vi "PH_O2_Watch.publish State.vi"(0 "i ref in":refnum<vi>, 5 "error in (no error)":errorcluster) -> (14 "i ref out":refnum<vi>, 19 "error out":errorcluster)   [LabVIEW 2014, in "PH_O2_Watch.lvlib"]
doc: "By this VI the device state is published via DIM service\n\nno info (0): no failure, prealert or alert, but at least one tag without info\non (2): no failure, prealert or alert, no limit set (\"99%\")\nfailure (3): failure\nalam (4): no failure, but alert\nStatus 1 (5): no alert or failure, but prealert\nStatus 2 (6): no failure, prealert or alert, and concentration smaller or equal than limit\nStatus 3 (7): no failure, prealert or alert, and concentration grater than limit"
uses:
  PH_O2_Watch.lvlib
  PH_Basics/PH_StatusHandler/PH_StatusHandler.Status.ctl
  PH_Basics/PH_StatusHandler/PH_StatusHandler.lvlib
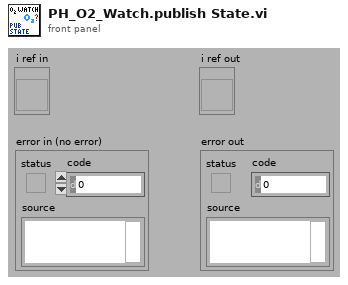
[diagram p1: front panel]
types:
  T1 = typedef "PH_StatusHandler.lvlib/PH_StatusHandler.Status.ctl" = i16
  T2 = typedef "PH_O2_Watch.lvlib/PH_O2_Watch.i attribute.ctl" = cluster{"GUI Refs":cluster{"PreAlert":refnum<vi>, "Alert":refnum<vi>, "Failure":refnum<vi>, "Concentration":refnum<vi>, "Delete":refnum<vi>, "Limit":refnum<vi>}, "State PreAlert":T1, "State Alert":T1, "State Failure":T1, "Concentration":dbl, "Limit":dbl}
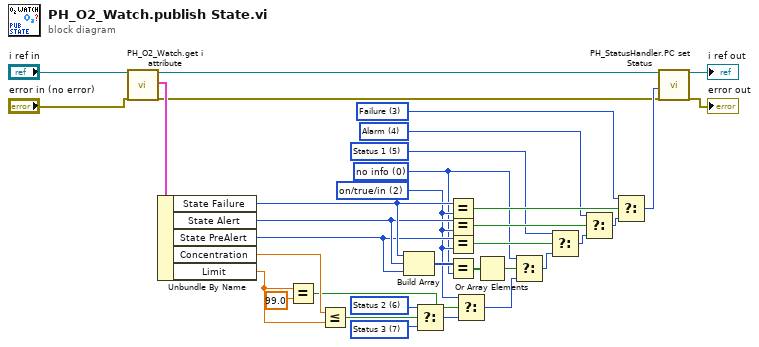
[diagram p0: block diagram]
diagram:
  w11 = T1 7 items=["no info", "off/false/out", "on/true/in", "Failure", "Alarm", "Status 1", "Status 2", "Status 3"] ("Status")
  w12 = T1 6 items=["no info", "off/false/out", "on/true/in", "Failure", "Alarm", "Status 1", "Status 2", "Status 3"] ("Status")
  w1 = T1 0 items=["no info", "off/false/out", "on/true/in", "Failure", "Alarm", "Status 1", "Status 2", "Status 3"] ("State Failure")
  w20 = T1 5 items=["no info", "off/false/out", "on/true/in", "Failure", "Alarm", "Status 1", "Status 2", "Status 3"] ("Status")
  w22 = T1 4 items=["no info", "off/false/out", "on/true/in", "Failure", "Alarm", "Status 1", "Status 2", "Status 3"] ("Status")
  w19 = T1 3 items=["no info", "off/false/out", "on/true/in", "Failure", "Alarm", "Status 1", "Status 2", "Status 3"] ("Status")
  w2 = T1 2 items=["no info", "off/false/out", "on/true/in", "Failure", "Alarm", "Status 1", "Status 2", "Status 3"] ("State Failure")
  n1 = call "PH_O2_Watch.get i attribute.vi"("i ref in"="i ref in", "error in (no error)"="error in (no error)") -> ("i ref out"=w32:refnum<vi>, "i attribute"=w31:T2, "error out"=w3:errorcluster)  [unwired: 15 in]
  n2 = Unbundle By Name(w31) -> ("State Failure"=w30:T1, "State Alert"=w29:T1, "State PreAlert"=w28:T1, "Concentration"=w27:dbl, "Limit"=w26:dbl)
  n3 = Equal?(x=w26, y=99.0) -> (x = y?=w9:bool)
  n4 = Less Or Equal?(x=w27, y=w26) -> (x <= y?=w13:bool)
  n5 = Build Array(w30, w29, w28) -> (w17:T1[])
  n6 = Select(t=w12, s=w13, f=w11) -> (s? t:f=w8:T1)
  n7 = Equal?(x=w30, y=w2) -> (x = y?=w25:bool)
  n8 = Equal?(x=w29, y=w2) -> (x = y?=w23:bool)
  n9 = Equal?(x=w28, y=w2) -> (x = y?=w18:bool)
  n10 = Equal?(x=w17, y=w1) -> (x = y?=w16:bool[])
  n11 = Select(t=w2, s=w9, f=w8) -> (s? t:f=w7:T1)
  n12 = Or Array Elements(Boolean array=w16) -> (logical OR=w14:bool)
  n13 = Select(t=w1, s=w14, f=w7) -> (s? t:f=w15:T1)
  n14 = Select(t=w20, s=w18, f=w15) -> (s? t:f=w21:T1)
  n15 = Select(t=w22, s=w23, f=w21) -> (s? t:f=w24:T1)
  n16 = Select(t=w19, s=w25, f=w24) -> (s? t:f=w4:T1)
  n17 = call "PH_StatusHandler.PC set Status.vi"("i ref in"=w32, "Status"=w4, "error in (no error)"=w3) -> ("i ref out"=→"i ref out":refnum<vi>, "error out"=→"error out":errorcluster)  [unwired: 15 in]
